vi "Raise_Lower_Value.vi"(9 "Raise Value?":bool, 11 "Value in":dbl) -> (3 "Value out":dbl)   [LabVIEW 2013]
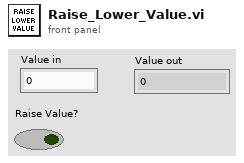
[diagram p1: front panel]
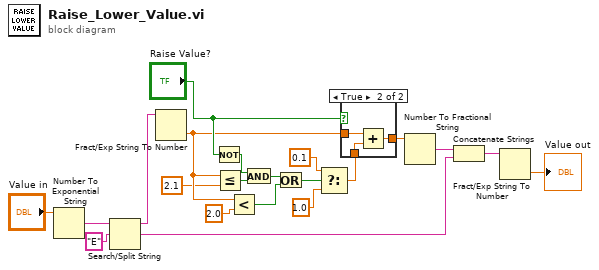
[diagram p0: block diagram]
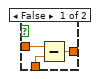
[diagram p2: hidden frame]
diagram:
  n1 = Number To Exponential String(number="Value in") -> (E-format string=w20:string)  [unwired: 3 in]
  n2 = Search/Split String(string=w20, search string/char (-)="E") -> (substring before match=w18:string, match + rest of string=w12:string)  [unwired: 1 in, 1 out]
  n3 = Fract/Exp String To Number(string=w18) -> (number=w3:dbl)  [unwired: 3 in, 1 out]
  n4 = Not(x="Raise Value?") -> (.not. x?=w8:bool)
  n5 = Less Or Equal?(x=w3, y=2.1) -> (x <= y?=w14:bool)
  n6 = Less?(x=w3, y=2.0) -> (x < y?=w5:bool)
  n7 = And(x=w8, y=w14) -> (x .and. y?=w6:bool)
  n8 = Or(x=w6, y=w5) -> (x .or. y?=w4:bool)
  n9 = Select(t=0.1, s=w4, f=1.0) -> (s? t:f=w16:dbl)
  n10 = case shown="True" "Raise Value?" {
    tunnel: w3 -> [w24 w26]
    tunnel: w16 -> [w23 w25]
    tunnel: [w22 w27] -> w13
    frame False {
      n11 = Subtract(x=w24, y=w23) -> (x-y=w22:dbl)
    }
    frame True {
      n12 = Add(x=w26, y=w25) -> (x+y=w27:dbl)
    }
  }
  n13 = Number To Fractional String(number=w13) -> (F-format string=w9:string)  [unwired: 3 in]
  n14 = Concatenate Strings(w9, w12) -> (w11:string)
  n15 = Fract/Exp String To Number(string=w11) -> (number=→"Value out":dbl)  [unwired: 3 in, 1 out]
